vi "模拟输入_连续(暂停触发）.vi"() -> ()   [LabVIEW 2013]
doc: "This example demonstrates how to acquire a continuous data."
uses:
  <userlib>/ArtDAQ/_SubVI/ArtDAQ_CreateAIVoltageChan.vi
  <userlib>/ArtDAQ/_SubVI/ArtDAQ_CfgSampClkTiming.vi
  <userlib>/ArtDAQ/_SubVI/ArtDAQ_CfgAnlgLvlPauseTrig.vi
  <userlib>/ArtDAQ/_SubVI/ArtDAQ_CfgDigLvlPauseTrig.vi
  <userlib>/ArtDAQ/_SubVI/ArtDAQ_CfgAnlgWindowPauseTrig.vi
  <userlib>/ArtDAQ/_SubVI/ArtDAQ_Read Analog DBL NChan NSamp.vi
panel:
  in  "触发模式":enum32{"模拟电平", "数字电平", "模拟窗"}(tab)
  in  "触发源":string(combo)="Dev1/ai0"
  in  "触发电平":dbl
  in  "触发条件":i32(ring)=10093 items=["高于电平"=10093, "低于电平"=10107]
  in  "触发源":string="/Dev1/PFI1"
  in  "触发条件":i32(ring)=10192 items=["高"=10192, "低"=10214]
  in  "窗顶部":dbl=0.5
  in  "窗底部":dbl
  in  "触发源":string(combo)="Dev1/ai0"
  in  "触发条件":i32(ring)=10199 items=["窗内"=10199, "窗外"=10251]
  in  "Stop":bool
  out "波形图":dbl[][](graph)
  in  "采样速率":dbl=10000.0 format="%#_13g"
  in  "每通道采样数":i32=1000
  in  "接线端配置":i32(ring)=-1 items=["默认"=-1, "单端"=10083, "非参考单端"=10078, "差分"=10106, "伪差分"=12529]
  in  "最小值(V)":dbl=-10.0 format="%#_13g"
  in  "最大值(V)":dbl=10.0 format="%#_13g"
  in  "物理通道":string(combo)="Dev2/ai0"
  out "错误":errorcluster
  # "通道属性"
  # "定时"
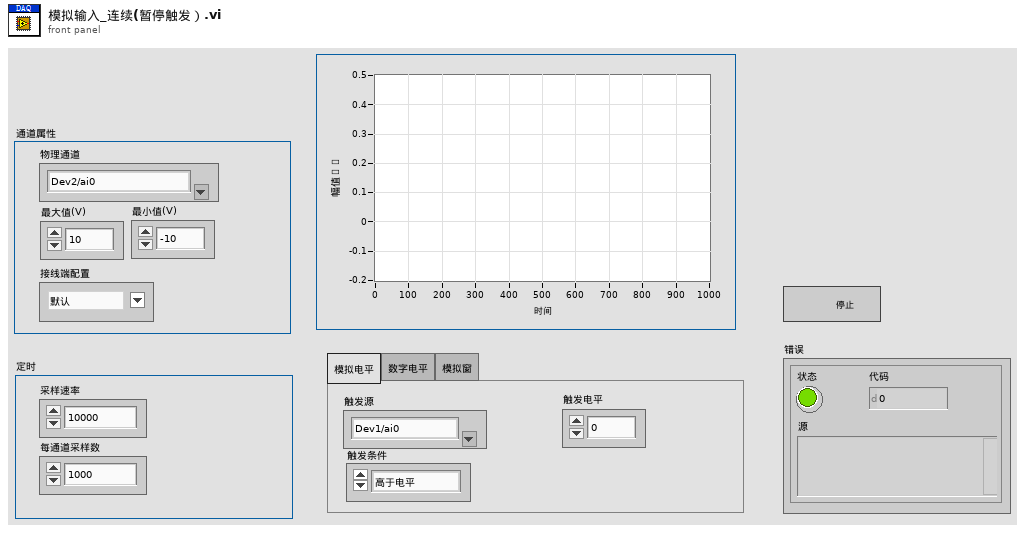
[diagram p1: front panel]
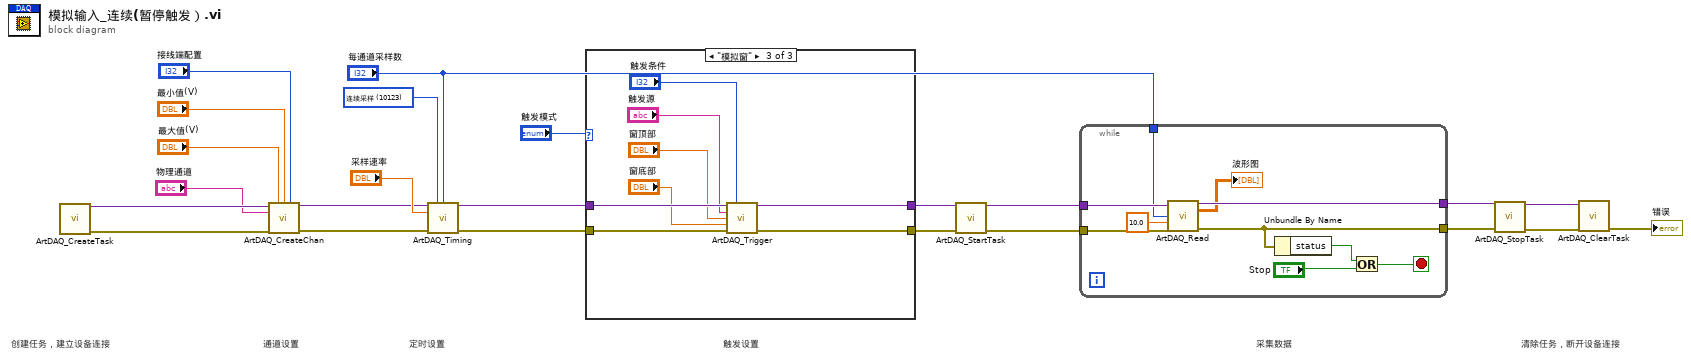
[diagram p0: block diagram]
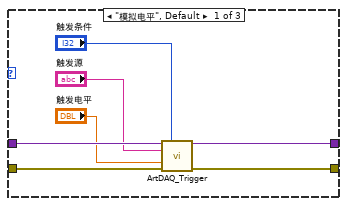
[diagram p2: hidden frame]
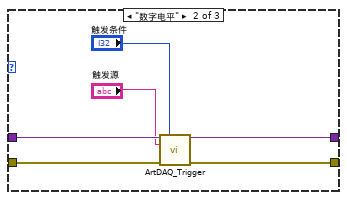
[diagram p3: hidden frame]
diagram:
  w18 = 10123 items=["有限点采样"=10178, "连续采样"=10123] ("SampleMode")
  # "清除任务，断开设备连接"
  # "采集数据"
  # "触发设置"
  # "定时设置"
  # "通道设置"
  # "创建任务，建立设备连接"
  n1 = call <userlib>:"ArtDAQ_CreateTask.vi"() -> ("任务句柄"=w12:variant, "错误输出"=w23:errorcluster)  [unwired: 14 in]
  n2 = call-poly <userlib>:"ArtDAQ_CreateChan.vi"("任务句柄"=w12, "最大值"="最大值(V)", "最小值"="最小值(V)", "接线端配置"="接线端配置", "物理通道"="物理通道", "错误输入"=w23) -> ("任务句柄"=w2:variant, "错误输出"=w19:errorcluster)  [unwired: 8 in]
  n3 = call-poly <userlib>:"ArtDAQ_Timing.vi"("任务句柄"=w2, "采样模式"=w18, "每通道采样数"="每通道采样数", "采样率"="采样速率", "错误输入"=w19) -> ("任务句柄"=w7:variant, "错误输出"=w5:errorcluster)  [unwired: 9 in]
  n4 = case shown="\"模拟窗\"" "触发模式" {
    tunnel: w7 -> [w30 w36 w44]
    tunnel: [w29 w35 w43] -> w6
    tunnel: w5 -> [w27 w34 w41]
    tunnel: [w28 w33 w42] -> w4
    frame "模拟电平", Default {
      n5 = call-poly <userlib>:"ArtDAQ_Trigger.vi"("任务句柄"=w30, "触发条件"="触发条件", "触发源"="触发源", "触发电平"="触发电平", "错误输入"=w27) -> ("任务句柄"=w29:variant, "错误输出"=w28:errorcluster)  [unwired: 9 in]
    }
    frame "数字电平" {
      n6 = call-poly <userlib>:"ArtDAQ_Trigger.vi"("任务句柄"=w36, "触发条件"="触发条件", "触发源"="触发源", "错误输入"=w34) -> ("任务句柄"=w35:variant, "错误输出"=w33:errorcluster)  [unwired: 10 in]
    }
    frame "模拟窗" {
      n7 = call-poly <userlib>:"ArtDAQ_Trigger.vi"("任务句柄"=w44, "触发条件"="触发条件", "触发源"="触发源", "窗顶部"="窗顶部", "窗底部"="窗底部", "错误输入"=w41) -> ("任务句柄"=w43:variant, "错误输出"=w42:errorcluster)  [unwired: 8 in]
    }
  }
  n8 = call <userlib>:"ArtDAQ_StartTask.vi"("任务句柄"=w6, "错误输入"=w4) -> ("任务句柄"=w15:variant, "错误输出"=w14:errorcluster)  [unwired: 12 in]
  n9 = while {
    tunnel: w15 -> [w54]
    tunnel: w14 -> [w53]
    tunnel: "每通道采样数" -> [w52]
    tunnel: [w50] -> w11
    tunnel: [w49] -> w10
    stop <- w47 stop-if-true
    n10 = call-poly <userlib>:"ArtDAQ_Read.vi"("任务句柄"=w54, "每通道采样数"=w52, "超时s"=10.0 ("Timeout"), "错误输入"=w53) -> ("任务句柄"=w50:variant, "数据"=→"波形图":dbl[][], "错误输出"=w49:errorcluster)  [unwired: 8 in, 1 out]
    n11 = Unbundle By Name(w49) -> ("status"=w48:bool)
    n12 = Or(x=w48, y="Stop") -> (x .or. y?=w47:bool)
  }
  n13 = call <userlib>:"ArtDAQ_StopTask.vi"("任务句柄"=w11, "错误输入"=w10) -> ("任务句柄"=w9:variant, "错误输出"=w8:errorcluster)  [unwired: 12 in]
  n14 = call <userlib>:"ArtDAQ_ClearTask.vi"("任务句柄"=w9, "错误输入"=w8) -> ("错误输出"=→"错误":errorcluster)  [unwired: 13 in]
